vi "xml_converter.vi"(0 "object":T1(array[cluster]), 5 "size":T2, 7 "folder":string="Funky Grooves", 9 "filename":string="Funky Grooves", 11 "XML File Path 2":path) -> ()   [LabVIEW 2021]
doc: "EasyXML Toolkit for LabVIEW version 3.0.0.170\nCopyright (c) 2016, JKI. All Rights Reserved."
panel:
  out "XML String":string
  in  "XML File Path":path
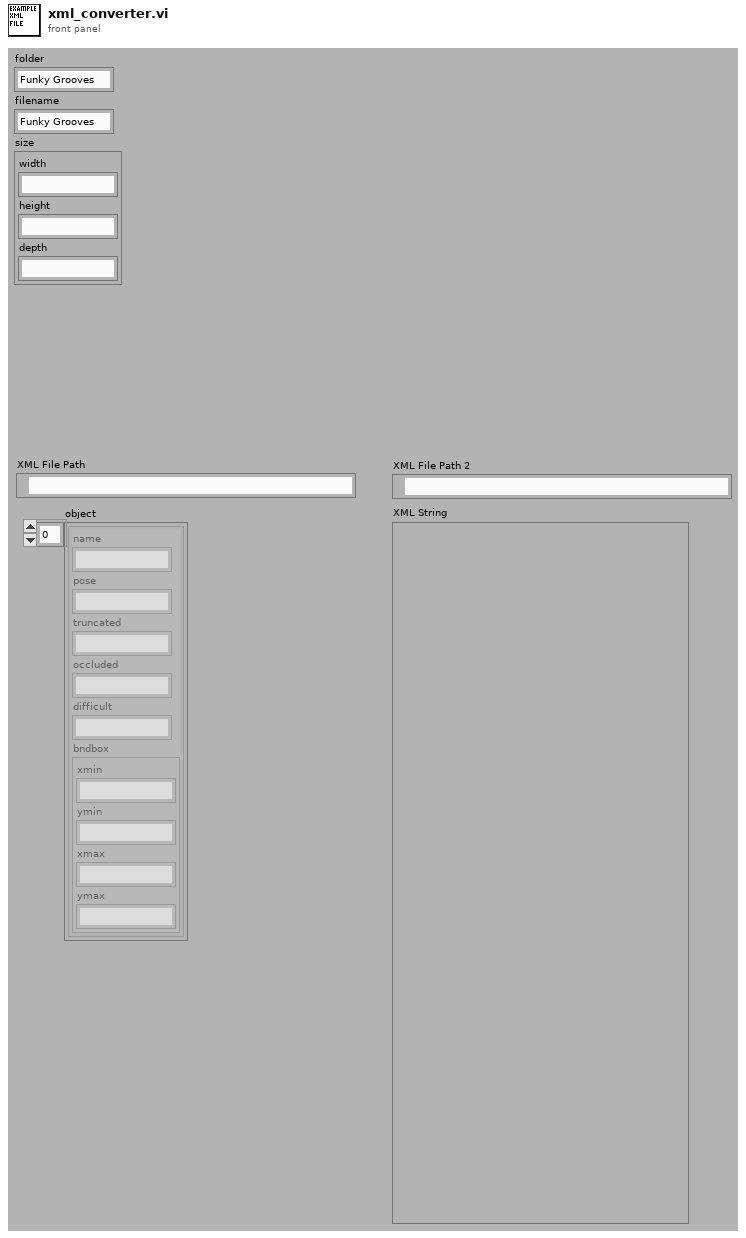
[diagram p1: front panel]
types:
  T1 = cluster{"name":string, "pose":string, "truncated":string, "occluded":string, "difficult":string, "bndbox":cluster{"xmin":string, "ymin":string, "xmax ":string, "ymax":string}}[]
  T2 = cluster{"width":string, "height":string, "depth ":string}
  T3 = cluster{"folder":string, "filename":string, "size":cluster{"width":string, "height":string, "depth ":string}, "object":cluster{"name":string, "pose":string, "truncated":string, "occluded":string, "difficult":string, "bndbox":cluster{"xmin":string, "ymin":string, "xmax ":string, "ymax":string}}[]}
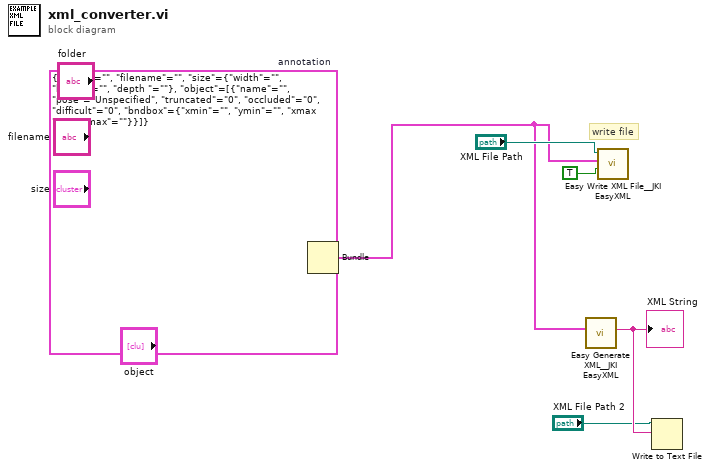
[diagram p0: block diagram]
diagram:
  w5 = T3 {"folder"="", "filename"="", "size"={"width"="", "height"="", "depth "=""}, "object"=[{"name"="", "pose"="Unspecified", "truncated"="0", "occluded"="0", "difficult"="0", "bndbox"={"xmin"="", "ymin"="", "xmax "="", "ymax"=""}}]}  # annotation
  # "write file"
  n1 = Bundle(cluster=w5, "folder"="folder", "filename"="filename", "size"="size", "object"="object") -> (w6:T3)
  n2 = call <vilib>:"Easy Generate XML__JKI EasyXML.vi"("LabVIEW Data"=w6) -> ("XML String"=w8:string)  [unwired: 9 in, 1 out]
  "XML String" <- w8
  n3 = call <vilib>:"Easy Write XML File__JKI EasyXML.vi"("Overwrite File? (false)"=TRUE, "LabVIEW Data"=w6, "XML File Path"="XML File Path") -> ()  [unwired: 7 in, 2 out]
  n4 = Write to Text File(file (use dialog)="XML File Path 2", text=w8) -> ()  [unwired: 2 in, 3 out]
